vi "Get Info.vi"(8 "error in (no error)":errorcluster, 11 "AAccount in":refnum<class "AAccount.lvclass">) -> (0 "error out":errorcluster, 2 "Account Information":T1, 3 "AAccount out":refnum<class "AAccount.lvclass">)   [LabVIEW 2020, in "AAccount.lvclass"]
uses:
  AAccount.lvclass
  Account Information STYP.ctl
  AAccount.lvclass/AAccount.ctl
  IInfoable/IInfoable.lvclass
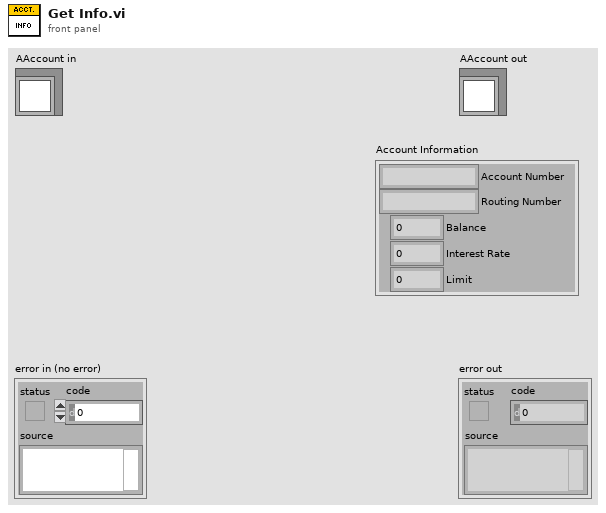
[diagram p1: front panel]
types:
  T1 = typedef "IInfoable.lvclass/Account Information STYP.ctl" = cluster{"Account Number":string, "Routing Number":string, "Balance":dbl, "Interest Rate":dbl, "Limit":dbl}
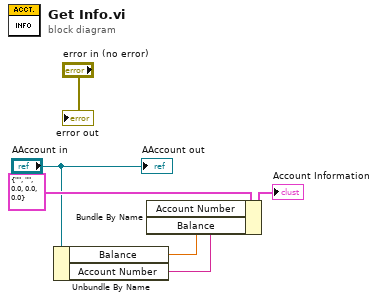
[diagram p0: block diagram]
diagram:
  n1 = Unbundle By Name("AAccount in") -> ("Balance"=w3:dbl, "Account Number"=w2:string)
  n2 = Bundle By Name(cluster=T1 {"Account Number"="", "Routing Number"="", "Balance"=0.0, "Interest Rate"=0.0, "Limit"=0.0} ("Account Information"), "Account Number"=w2, "Balance"=w3) -> (→"Account Information":T1)
  "error out" <- "error in (no error)"
  "AAccount out" <- "AAccount in"
